vi "LJStreamM write to file.vi"(0 "Data File Reference In":path, 1 "Working Directory":path, 2 "Starting #":u32, 3 "Channel Names":string[](array[string]), 4 "Raw Value":dbl[][](array[numeric]), 5 "Scaled Data":dbl[][](array[numeric]) format="%.3f", 6 "Data File Prefix":string, 7 "Scan Rate":dbl=50.0 format="%.2f", 9 "Max File Size (Bytes)":i32, 11 "Starting Scan Time":dbl format="%.2f", 12 "Disable Scaling":bool, 13 "Write to file?":bool) -> (14 "Data File Reference Out":path, 15 "Working Directory Out":path, 16 "Data File #":u32)   [LabVIEW 2026]
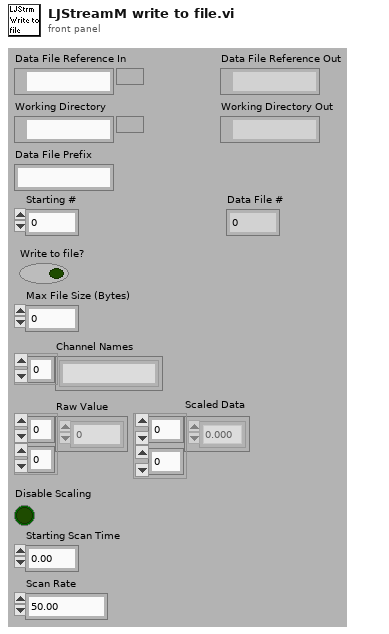
[diagram p1: front panel]
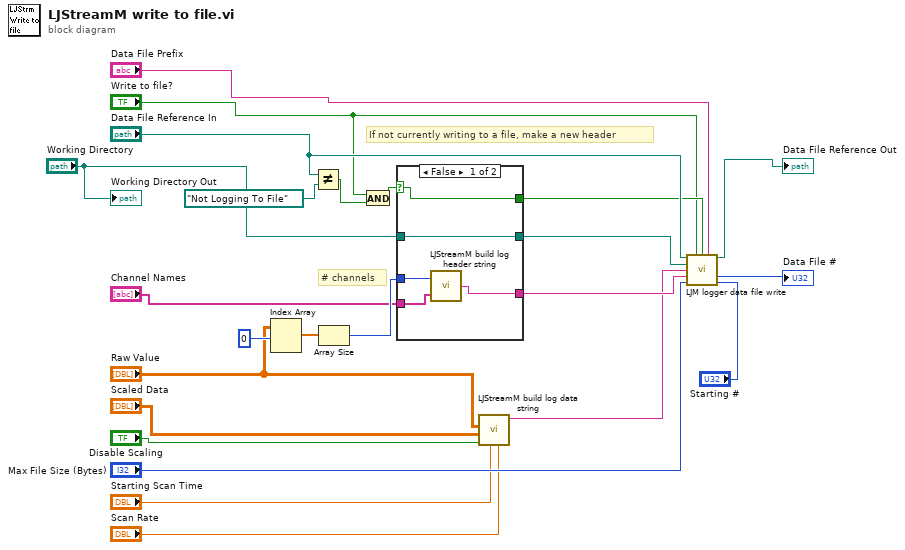
[diagram p0: block diagram]
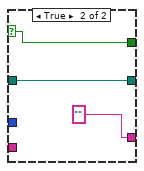
[diagram p2: hidden frame]
diagram:
  # "# channels"
  # "If not currently writing to a file, make a new header"
  n1 = Index Array(array="Raw Value", index (row)=0 ("index")) -> (element=w8:dbl[])  [unwired: 1 in]
  n2 = Not Equal?(x="Data File Reference In", y=path "Not Logging To File") -> (x != y?=w5:bool)
  n3 = Array Size(array=w8) -> (size(s)=w15:i32)
  n4 = And(x="Write to file?", y=w5) -> (x .and. y?=w3:bool)
  n5 = case shown="False" w3 {
    selector: w3 -> [w29 w32]
    tunnel: [w27 "" ("Header String")] -> w19
    tunnel: [w29 w32] -> w17
    tunnel: "Working Directory" -> [w28 w30]
    tunnel: [w28 w30] -> w16
    tunnel: w15 -> [w26 _]
    tunnel: "Channel Names" -> [w25 _]
    frame False {
      n6 = call "LJStreamM build log header string.vi"("Names"=w25, "# Channels"=w26) -> ("Header String"=w27:string)
    }
    frame True {
    }
  }
  n7 = call "LJStreamM build log data string.vi"("Scan Rate"="Scan Rate", "Time"="Starting Scan Time", "Disable Scaling"="Disable Scaling", "Scaled Data"="Scaled Data", "Raw Data"="Raw Value") -> ("Output data"=w13:string)  [unwired: 6 in]
  n8 = call "LJM logger data file write.vi"("Current Data File In"="Data File Reference In", "Write To File"="Write to file?", "Currently Writing"=w17, "Data File Prefix"="Data File Prefix", "Working Directory"=w16, "Log data"=w13, "Header String"=w19, "max file size (bytes)"="Max File Size (Bytes)", "Starting #"="Starting #") -> ("Current Data File Out"=→"Data File Reference Out":path, "Data File #"=→"Data File #":u32)  [unwired: 5 in]
  "Working Directory Out" <- "Working Directory"
